vi "InitSessionCfg.vi"(8 "error in (no error)":errorcluster, 11 "This VI":refnum<vi>) -> (0 "error out":errorcluster, 3 "Showagian 2":bool)   [LabVIEW 2019]
panel:
  in  "Showagian":bool
  in  "Skip":bool caption="Load"
  in  "Load":bool
  in  "String":string="Please load a valid session:"
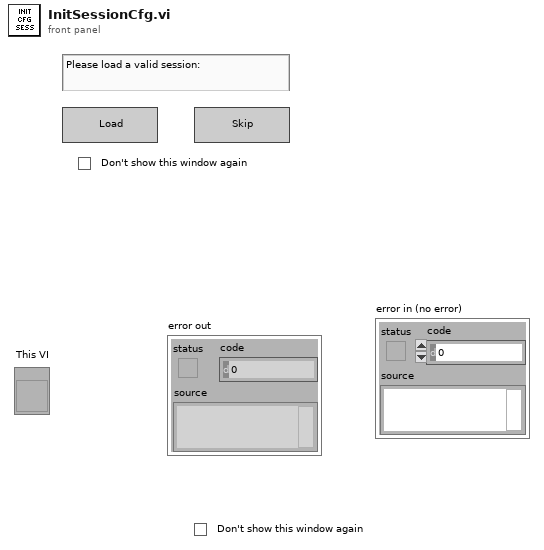
[diagram p1: front panel]
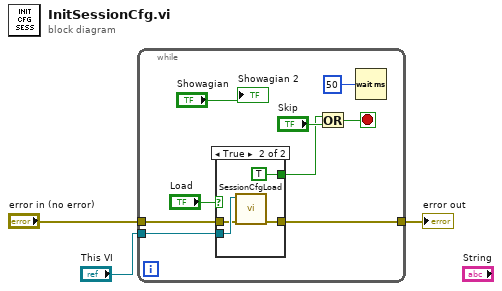
[diagram p0: block diagram]
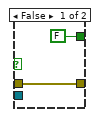
[diagram p2: hidden frame]
diagram:
  n1 = while {
    tunnel: "This VI" -> [w10]
    tunnel: "error in (no error)" -> [w9]
    tunnel: [w8] -> w1
    stop <- w7 stop-if-true
    n2 = case shown="True" "Load" {
      tunnel: w10 -> [_ w18]
      tunnel: w9 -> [w14 w17]
      tunnel: [w14 w16] -> w8
      tunnel: [FALSE TRUE] -> w5
      frame False {
      }
      frame True {
        n3 = call "SessionCfgLoad.vi"("error in (no error)"=w17, "This VI"=w18) -> ("error out"=w16:errorcluster)  [unwired: 9 in]
      }
    }
    n4 = Or(x=w5, y="Skip") -> (x .or. y?=w7:bool)
    n5 = Wait (ms)(milliseconds to wait=u32 50) -> ()  [unwired: 1 out]
    "Showagian 2" <- "Showagian"
  }
  "error out" <- w1
